vi "Tell Controller to Launch Settings Dialog.vi"(8 "error in (no error)":errorcluster, 11 "UI in":refnum<class "UI.lvclass">) -> (0 "error out":errorcluster, 3 "UI out":refnum<class "UI.lvclass">)   [LabVIEW 2016, in "Measurement UI.lvlib" / "Measurement UI.lvclass"]
uses:
  Msmt UI/Measurement UI.lvclass
  UI.lvclass
  C:/Program Files (x86)/National Instruments/LabVIEW 2016/vi.lib/ActorFramework/Actor/Actor.lvclass
  <vilib>/ActorFramework/Actor/Actor.lvclass/Actor.ctl
  <vilib>/ActorFramework/Message Enqueuer/Message Enqueuer.lvclass/Message Enqueuer.ctl
  <vilib>/ActorFramework/Message Enqueuer/Enqueue.vi
  Controller/Messages/Launch Settings Dialog Msg/Launch Settings Dialog Msg.lvclass
  C:/Program Files (x86)/National Instruments/LabVIEW 2016/vi.lib/ActorFramework/Message/Message.lvclass
  <vilib>/ActorFramework/Message Priority Queue/Priority Enqueue.vi
  <vilib>/ActorFramework/Actor/Actor.lvclass
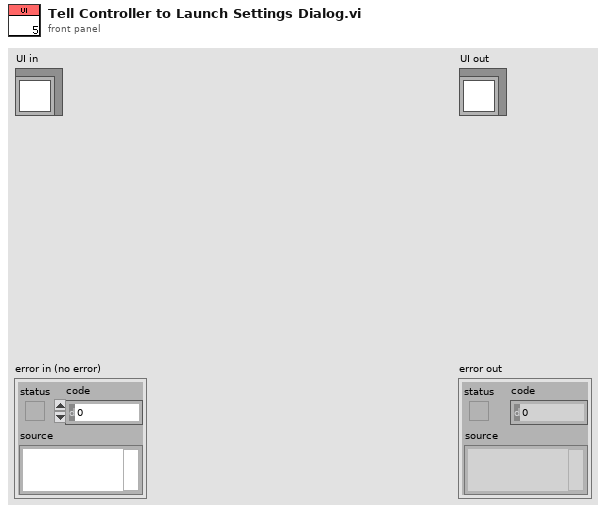
[diagram p1: front panel]
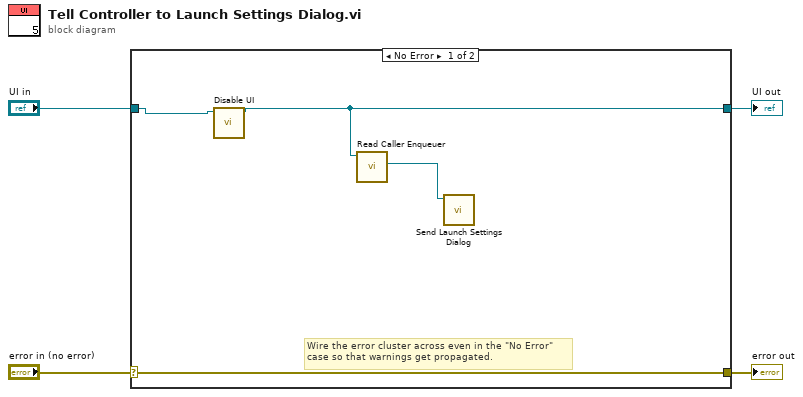
[diagram p0: block diagram]
diagram:
  n1 = case shown="No Error" "error in (no error)" {
    selector: "error in (no error)" -> [w8 w10]
    tunnel: [w8 w10] -> w3
    tunnel: [w5 w9] -> w1
    tunnel: "UI in" -> [w6 w9]
    frame No Error {
      # "Wire the error cluster across even in the \"No Error\"\ncase so that warnings get propagated."
      n2 = call-dynamic "Disable UI.vi"("UI in"=w6) -> ("UI out"=w5:refnum<class "UI.lvclass">)  [unwired: 9 in, 1 out]
      n3 = call <vilib>:"Read Caller Enqueuer.vi"("Actor"=w5) -> ("Caller Enqueuer"=w7:refnum<class "Message Enqueuer.lvclass">)  [unwired: 10 in]
      n4 = call "Send Launch Settings Dialog.vi"("Message Enqueuer"=w7) -> ()  [unwired: 9 in, 2 out]
    }
    frame Error {
    }
  }
  "error out" <- w3
  "UI out" <- w1
